vi "FTW-CodeGen-Initialize.vi"(5 "XRef":refnum<vi>) -> (4 "State Out":T1={"Terminal Type"=variant(string ""), "PathWired"=FALSE})   [LabVIEW 2014, in "FTW-JSON-Fetch.xnode"]
uses:
  FTW-JSON-Fetch.xnode
  FTW-CodeGen-State.ctl
panel:
  # "Inputs"
  # "Outputs"
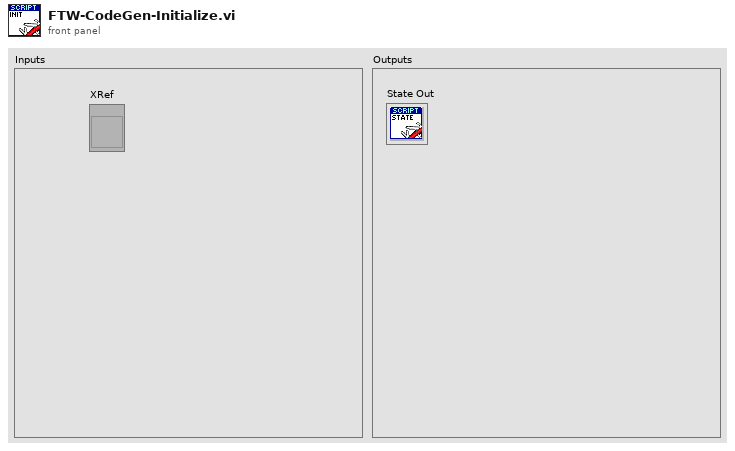
[diagram p1: front panel]
types:
  T1 = typedef "FTW-JSON-Fetch.xnode/FTW-CodeGen-State.ctl" = cluster{"Terminal Type":variant, "PathWired":bool}
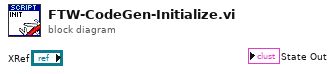
[diagram p0: block diagram]
diagram:
